vi "Export config to file.vi"(8 "error in (no error)":errorcluster, 11 "Node Ptr":u64 format="%.0x") -> (0 "error out":errorcluster)   [LabVIEW 2017, in "Shared Variables CD 2.0 Configuration.lvlib"]
uses:
  Shared Variables CD 2.0 Configuration.lvlib
  Public/Documents/National Instruments/NI VeriStand 2017/Custom Devices/Shared Variables CD 2.0/Data/ImportExport.lvlibp/Operation.ctl
  Public/Documents/National Instruments/NI VeriStand 2017/Custom Devices/Shared Variables CD 2.0/Data/Channel.lvlibp/Channel.lvclass
  Support/ChannelVS/ChannelVS.lvclass
  C:/Users/Public/Documents/National Instruments/NI VeriStand 2017/Custom Devices/Shared Variables CD 2.0/Data/Channel.lvlibp/Channel.lvclass
  Shared/SV Global.vi
  <vilib>/NI VeriStand/Custom Device API/Custom Device API.lvlib
  Public/Documents/National Instruments/NI VeriStand 2017/Custom Devices/Shared Variables CD 2.0/Data/ImportExport.lvlibp
panel:
  in  "Tag":string
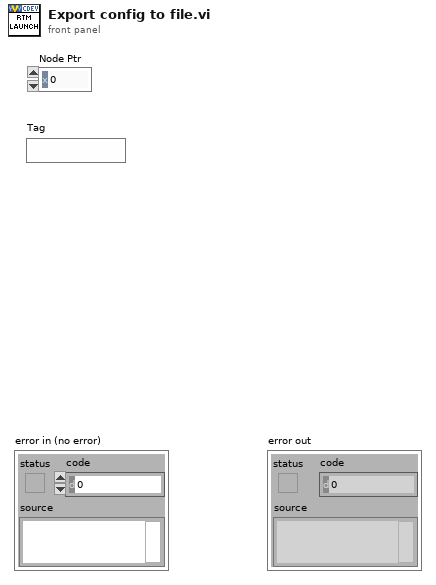
[diagram p1: front panel]
types:
  T1 = typedef "ImportExport.lvlibp/Operation.ctl" = enum16{"Import", "Export"}
  T2 = typedef "Custom Device API.lvlib/Custom Device Item Ref.ctl" = u64
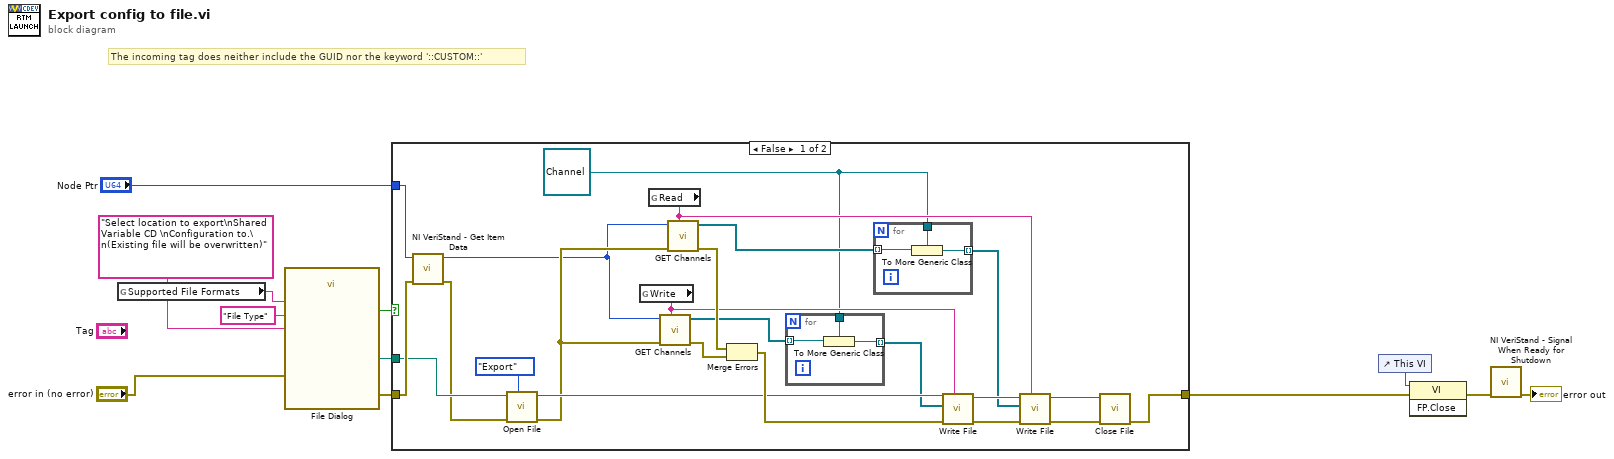
[diagram p0: block diagram]
diagram:
  # "The incoming tag does neither include the GUID nor the keyword '::CUSTOM::'"
  n1 = global read "SV Global.vi" "Supported File Formats"() -> (w1:string)
  n2 = call "File Dialog"("prompt"="Select location to export\nShared Variable CD \nConfiguration to.\n(Existing file will be overwritten)", "error in"="error in (no error)", "pattern (all files)"=w1, "pattern label"="File Type") -> ("selected path"=w6:path, "cancelled"=w7:bool, "error out"=w4:errorcluster)  [unwired: 8 in, 1 out]
  n3 = case shown="False" w7 {
    tunnel: "Node Ptr" -> [w35 _]
    tunnel: w4 -> [w34 w42]
    tunnel: [w26 w42] -> w8
    tunnel: w6 -> [w33 _]
    frame False {
      w15 = refnum<class "Channel.lvclass"> refnum ("Channel.lvlibp:Channel.lvclass")
      n4 = call <vilib>:"NI VeriStand - Get Item Data.vi"("error in (no error)"=w34, "Item Ref in"=w35) -> ("error out"=w32:errorcluster, "Item Ref out"=w20:T2)  [unwired: 6 in, 2 out]
      n5 = call "Open File.vi"("Operation"=Operation."Export", "error in (no error)"=w32, "Path"=w33) -> ("error out"=w21:errorcluster, "ConfigFile out"=w29:refnum<class "ConfigFile.lvclass">)  [unwired: 7 in]
      n6 = global read "SV Global.vi" "Write"() -> (w19:string)
      n7 = global read "SV Global.vi" "Read"() -> (w18:string)
      n8 = call "GET Channels.vi"("Channel Direction"=w19, "error in (no error)"=w21, "Item Ref in"=w20) -> ("error out"=w22:errorcluster, "VS Channel Array"=w16:refnum<class "ChannelVS.lvclass">[])  [unwired: 7 in]
      n9 = call "GET Channels.vi"("Channel Direction"=w18, "error in (no error)"=w21, "Item Ref in"=w20) -> ("error out"=w23:errorcluster, "VS Channel Array"=w17:refnum<class "ChannelVS.lvclass">[])  [unwired: 7 in]
      n10 = Merge Errors(w23, w22) -> (w31:errorcluster)
      n11 = for {
        tunnel: w16 -> [w38] mode=indexing
        tunnel: w15 -> [w37]
        tunnel: [w36] -> w14 mode=indexing
        n12 = To More Generic Class(target class=w37, reference=w38) -> (generic class reference=w36:refnum<class "Channel.lvclass">)
      }
      n13 = for {
        tunnel: w17 -> [w41] mode=indexing
        tunnel: w15 -> [w40]
        tunnel: [w39] -> w13 mode=indexing
        n14 = To More Generic Class(target class=w40, reference=w41) -> (generic class reference=w39:refnum<class "Channel.lvclass">)
      }
      n15 = call "Write File.vi"("Channel Direction"=w19, "error in (no error)"=w31, "Channels"=w14, "ConfigFile in"=w29) -> ("error out"=w30:errorcluster, "ConfigFile out"=w28:refnum<class "ConfigFile.lvclass">)  [unwired: 6 in]
      n16 = call "Write File.vi"("Channel Direction"=w18, "error in (no error)"=w30, "Channels"=w13, "ConfigFile in"=w28) -> ("error out"=w27:errorcluster, "ConfigFile out"=w25:refnum<class "ConfigFile.lvclass">)  [unwired: 6 in]
      n17 = call "Close File.vi"("error in (no error)"=w27, "ConfigFile in"=w25) -> ("error out"=w26:errorcluster)  [unwired: 9 in]
    }
    frame True {
    }
  }
  n18 = control-ref of="This VI"() -> (w10:refnum<vi>)
  n19 = invoke class="VI" method="FP.Close"(reference=w10, error in=w8) -> (error out=w9:errorcluster)  [unwired: 1 in, 2 out]
  n20 = call <vilib>:"NI VeriStand - Signal When Ready for Shutdown.vi"("error in (no error)"=w9) -> ("error out"=→"error out":errorcluster)  [unwired: 10 in]
